vi "ZC_status.vi"(3 "key":string, 7 "LabVIEW Web Service Request":refnum<class "Web Request.lvclass"> caption="LabVIEW Web服务请求", 8 "number":string, 9 "name":string, 10 "id":string, 11 "action":string) -> (0 "error":errorcluster)   [LabVIEW 2017]
uses:
  <vilib>/wsapi/Web Request.lvclass
panel:
  out "postdata":string caption="post数据"
  out "error out":errorcluster caption="错误输出"
  # "Web服务请求输入接线端用于调用“Web服务”选板的VI。除非不需要访问该选板，否则不要在连线板上删除这个输入接线端。"
  # "添加至连线板的每一个其他输入控件，在URL中对应于一个输入。如需在接线端模式输出（默认设置）下包含显示控件，则该显示控件必须与连线板相连。"
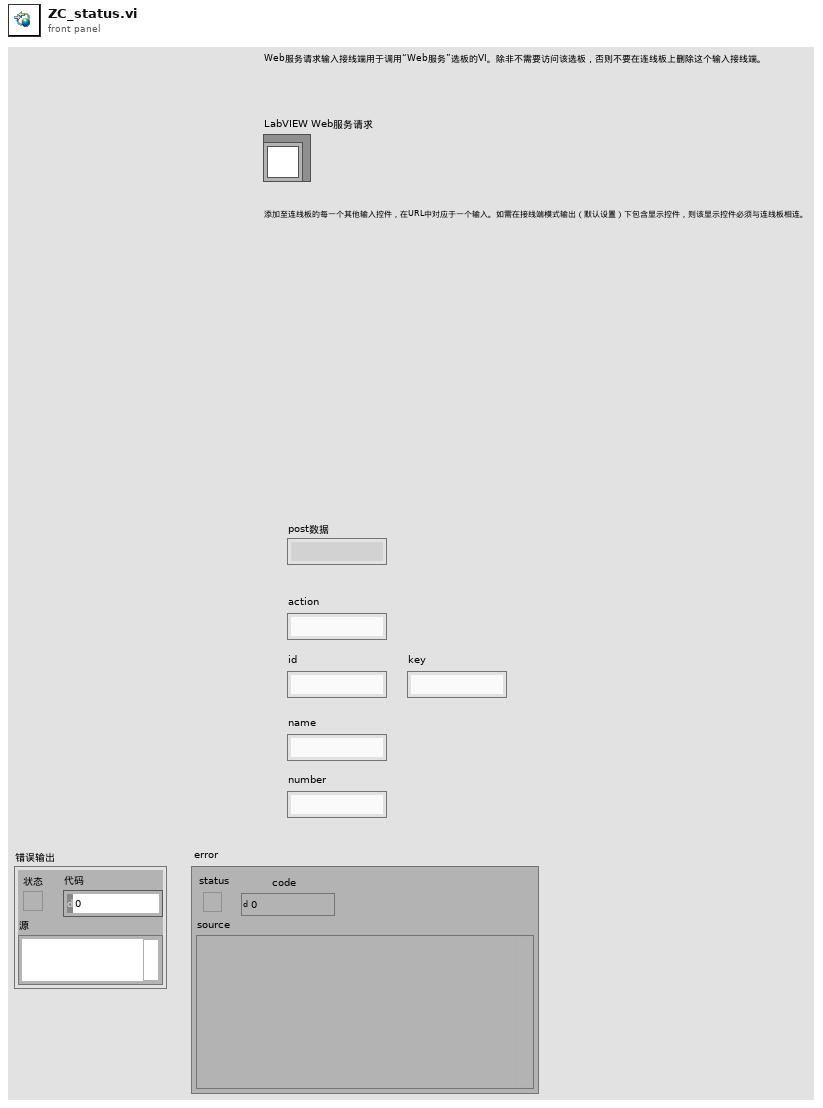
[diagram p1: front panel]
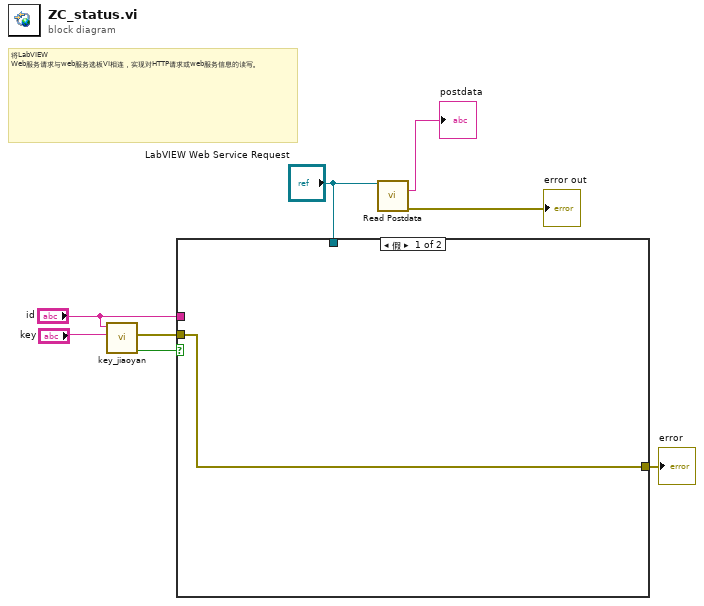
[diagram p0: block diagram]
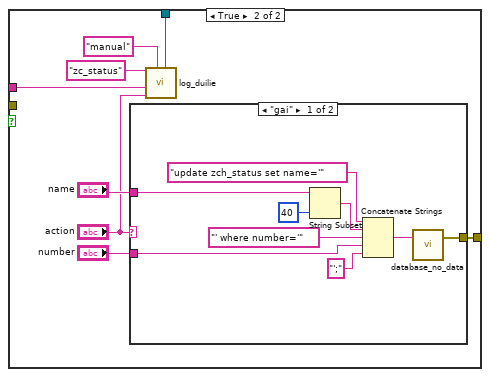
[diagram p2: hidden frame]
diagram:
  # "将LabVIEW Web服务请求与web服务选板VI相连，实现对HTTP请求或web服务信息的读写。"
  n1 = call "key_jiaoyan.vi"("key_client"="key", "gonghao"="id") -> ("jy"=w2:bool, "error"=w1:errorcluster)  [unwired: 8 in]
  n2 = case shown="假" w2 {
    tunnel: [w9 w17] -> w7
    tunnel: "LabVIEW Web Service Request" -> [_ w12]
    tunnel: "id" -> [_ w10]
    tunnel: w1 -> [w9 _]
    frame False {
    }
    frame True {
      n3 = case shown="\"gai\"" "action" {
        tunnel: [w22 _] -> w17
        tunnel: "name" -> [w21 _]
        tunnel: "number" -> [w19 _]
        frame "gai" {
          n4 = String Subset(string=w21, length (rest)=40 ("长度（剩余）")) -> (substring=w25:string)  [unwired: 1 in]
          n5 = Concatenate Strings("update zch_status set name='" ("格式字符串"), w25, "' where number='" ("字符串"), w19, "';" ("字符串")) -> (w26:string)
          n6 = call "database_no_data.vi"("input"=w26) -> ("error"=w22:errorcluster)  [unwired: 2 in]
        }
        frame Default {
        }
      }
      n7 = call "log_duilie.vi"("LabVIEW Web Service Request"=w12, "type"="manual", "action"="action", "user"=w10, "yw"="zc_status") -> ()  [unwired: 7 in]
    }
  }
  "error" <- w7
  n8 = call <vilib>:"Read Postdata.vi"("LabVIEW Web Service Request"="LabVIEW Web Service Request") -> ("postdata"=→"postdata":string, "error out"=→"error out":errorcluster)  [unwired: 12 in, 1 out]
